vi "Handle Messages.vi"(8 "error in (no error)":errorcluster, 9 "Message Data":variant, 10 "Message":string, 11 "Thermal Chamber Controller In":refnum<class "Thermal Chamber Controller.lvclass">) -> (0 "error out":errorcluster, 3 "Thermal Chamber Controller Out":refnum<class "Thermal Chamber Controller.lvclass">)   [LabVIEW 2020, in "Thermal Chamber Controller.lvclass"]
uses:
  Thermal Chamber Controller.lvclass
  C:/Program Files (x86)/National Instruments/LabVIEW 2020/vi.lib/Astemes/Triarc Framework/Helper Loop/Helper Loop.lvclass
  C:/Program Files (x86)/National Instruments/LabVIEW 2020/vi.lib/Astemes/Triarc Framework/Process/Process.lvclass
  <vilib>/Astemes/Triarc Framework/Process/Process.lvclass/Process.ctl
  Thermal Chamber Controller.lvclass/Thermal Chamber Controller.ctl
  Thermal Chamber Response Simlator/Thermal Chamber Response Simlator.lvclass/Thermal Chamber Response Simlator.ctl
  Private/Heater State.ctl
  <vilib>/Astemes/Triarc Framework/Process/Public/Lifecycle/Get Lifecycle State.vi
  <vilib>/Astemes/Triarc Framework/Process/Public/Broadcasting/Register for Broadcast Events.vi
  <vilib>/Astemes/Triarc Framework/Broadcast Event Helpers/Dequeue Broadcast Message by Message.vi
  <vilib>/Astemes/Triarc Framework/Process/Private/SubVIs/Handle Debug Data.vi
  <vilib>/Utility/error.llb/Clear Errors.vi
  <vilib>/Astemes/Triarc Framework/Broadcast Event Helpers/Execution timer.vi
  <vilib>/Utility/High Resolution Relative Seconds.vi
  <vilib>/Utility/error.llb/Error Cluster From Error Code.vi
  <vilib>/Astemes/Triarc Framework/Broadcast Event Helpers/Dequeue Broadcast Message.vi
  Thermal Chamber Response Simlator/Private/Get Current Time if Not Set.vi
  Thermal Chamber Response Simlator/Get Actual Temperature.vi
  <vilib>/Astemes/Triarc Framework/Process/Process.lvclass
  <vilib>/Astemes/Triarc Framework/View/View.lvclass
  <vilib>/Astemes/Triarc Framework/Helper Loop/Helper Loop.lvclass
  Thermal Chamber Response Simlator/Thermal Chamber Response Simlator.lvclass
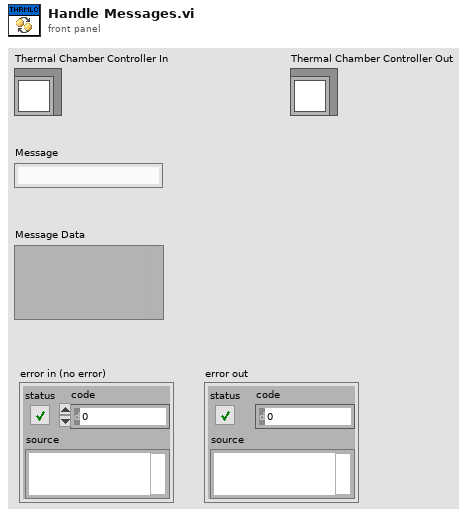
[diagram p1: front panel]
types:
  T1 = typedef "Thermal Chamber Controller.lvclass/Heater State.ctl" = enum16{"Heater Disabled", "Heater Enabled"}
  T2 = typedef "Thermal Chamber Controller.lvclass/Chamber State.ctl" = cluster{"Actual Temperature":dbl, "Temperature Set Point":dbl, "Temperature Ramp Rate":dbl, "Heater State":T1}
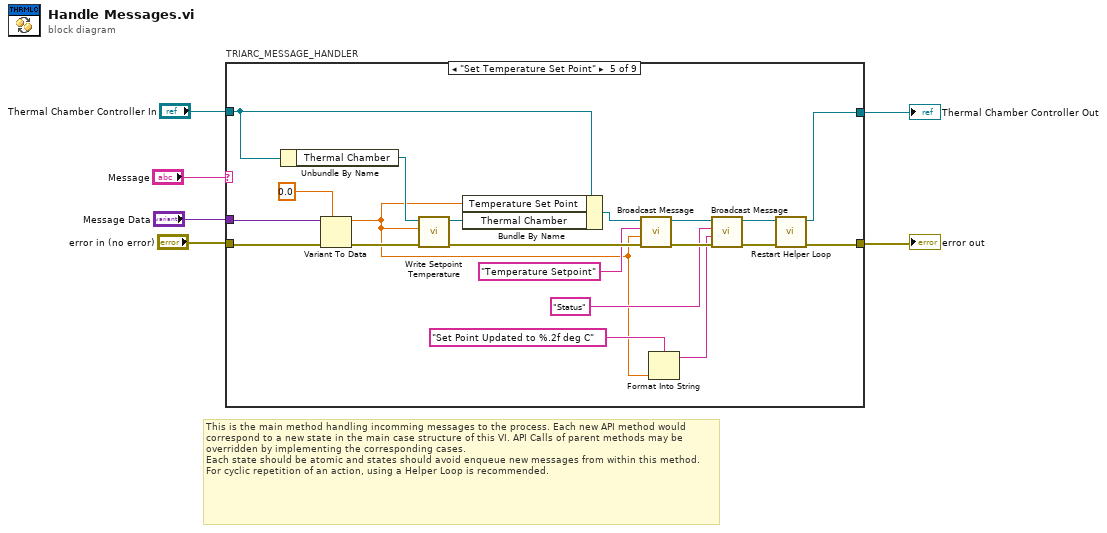
[diagram p0: block diagram]
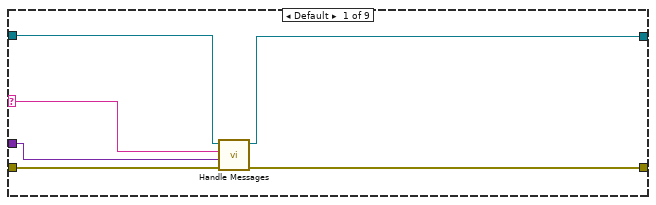
[diagram p2: hidden frame]
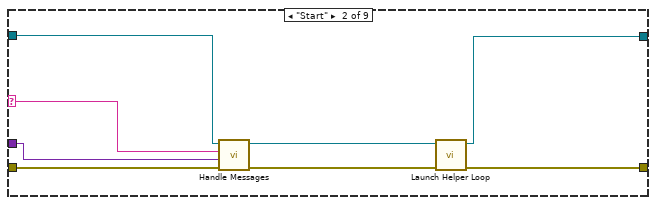
[diagram p3: hidden frame]
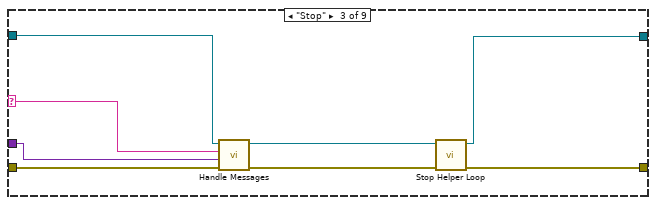
[diagram p4: hidden frame]
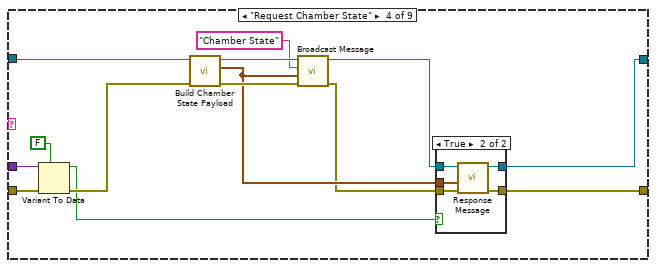
[diagram p5: hidden frame]
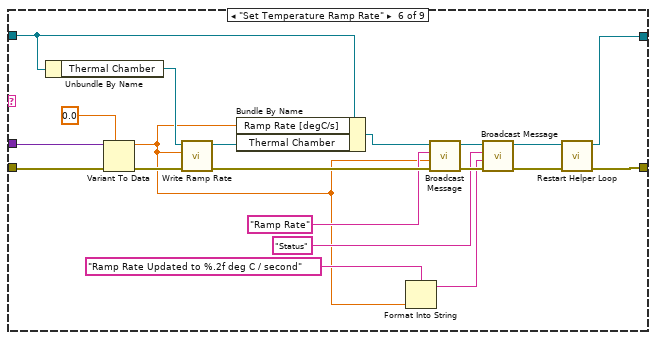
[diagram p7: hidden frame]
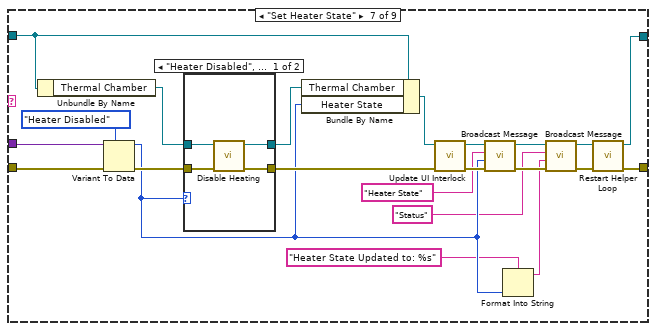
[diagram p8: hidden frame]
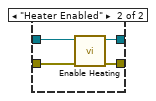
[diagram p9: hidden frame]
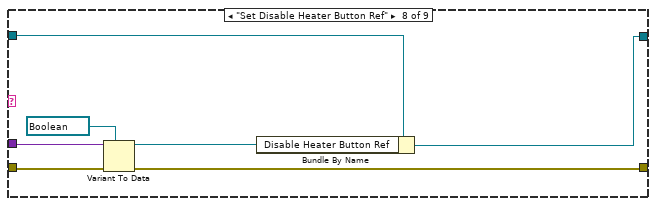
[diagram p10: hidden frame]
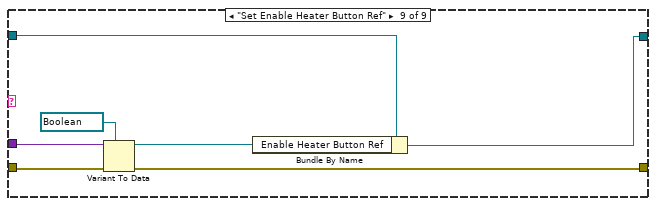
[diagram p11: hidden frame]
diagram:
  # "This is the main method handling incomming messages to the process. Each new API method would correspond to a new state in the main case structure of this VI. API Calls of parent methods may be overridden by implementing the corresponding cases.\nEach state should be atomic and states should avoid enqueue new messages from within this method. For cyclic repetition of an action, using a Helper Loop is recommended."
  n1 = case "TRIARC_MESSAGE_HANDLER" shown="\"Set Temperature Set Point\"" "Message" {
    selector: "Message" -> [w10 w18 w26 _ _ _ _ _ _]
    tunnel: "error in (no error)" -> [w9 w17 w25 w42 w69 w89 w111 w126 w133]
    tunnel: "Thermal Chamber Controller In" -> [w12 w20 w28 w37 w65 w86 w107 w125 w132]
    tunnel: "Message Data" -> [w11 w19 w27 w41 w67 w88 w109 w122 w128]
    tunnel: [w8 w13 w21 w39 w52 w72 w92 w123 w130] -> w2
    tunnel: [w7 w15 w23 w38 w50 w70 w90 w124 w131] -> w1
    frame Default {
      n2 = call-parent "Handle Messages.vi"("error in (no error)"=w9, "Message Data"=w11, "Message"=w10, "View In"=w12) -> ("error out"=w8:errorcluster, "View Out"=w7:refnum<class "Thermal Chamber Controller.lvclass">)  [unwired: 6 in]
    }
    frame "Start" {
      n3 = call-parent "Handle Messages.vi"("error in (no error)"=w17, "Message Data"=w19, "Message"=w18, "View In"=w20) -> ("error out"=w14:errorcluster, "View Out"=w16:refnum<class "Thermal Chamber Controller.lvclass">)  [unwired: 6 in]
      n4 = call <vilib>:"Launch Helper Loop.vi"("error in (no error)"=w14, "Helper Loop In"=w16) -> ("error out"=w13:errorcluster, "Helper Loop Out"=w15:refnum<class "Thermal Chamber Controller.lvclass">)  [unwired: 8 in]
    }
    frame "Stop" {
      n5 = call-parent "Handle Messages.vi"("error in (no error)"=w25, "Message Data"=w27, "Message"=w26, "View In"=w28) -> ("error out"=w22:errorcluster, "View Out"=w24:refnum<class "Thermal Chamber Controller.lvclass">)  [unwired: 6 in]
      n6 = call <vilib>:"Stop Helper Loop.vi"("error in (no error)"=w22, "Helper Loop In"=w24) -> ("error out"=w21:errorcluster, "Helper Loop Out"=w23:refnum<class "Thermal Chamber Controller.lvclass">)  [unwired: 7 in, 1 out]
    }
    frame "Request Chamber State" {
      n7 = Variant To Data(error in=w42, type=FALSE, Variant=w41) -> (data=w31:bool, error out=w35:errorcluster)
      n8 = call "Build Chamber State Payload.vi"("error in (no error)"=w35, "Thermal Chamber Controller In"=w37) -> ("error out"=w36:errorcluster, "Chamber State Payload"=w32:T2, "Thermal Chamber Controller Out"=w34:refnum<class "Thermal Chamber Controller.lvclass">)  [unwired: 7 in]
      n9 = call-dynamic "Broadcast Message.vi"("error in (no error)"=w36, "Message Data"=w32, "Message"="Chamber State", "Process In"=w34) -> ("error out"=w29:errorcluster, "Process Out"=w30:refnum<class "Thermal Chamber Controller.lvclass">)  [unwired: 6 in]
      n10 = case shown="True" w31 {
        tunnel: [w43 w49] -> w39
        tunnel: [w44 w48] -> w38
        tunnel: w29 -> [w43 w47]
        tunnel: w30 -> [w44 w46]
        tunnel: w32 -> [_ w45]
        frame False {
        }
        frame True {
          n11 = call <vilib>:"Response Message.vi"("error in (no error)"=w47, "Response Message Data"=w45, "Process In"=w46) -> ("error out"=w49:errorcluster, "Process Out"=w48:refnum<class "Thermal Chamber Controller.lvclass">)  [unwired: 7 in]
        }
      }
    }
    frame "Set Temperature Set Point" {
      n12 = Unbundle By Name(w65) -> ("Thermal Chamber"=w63:refnum<class "Thermal Chamber Response Simlator.lvclass">)
      n13 = Variant To Data(error in=w69, type=0.0 ("Numeric"), Variant=w67) -> (data=w54:dbl, error out=w68:errorcluster)
      n14 = call "Write Setpoint Temperature.vi"("error in (no error)"=w68, "Setpoint Temperature [degC]"=w54, "Thermal Chamber Response Simlator In"=w63) -> ("error out"=w64:errorcluster, "Thermal Chamber Response Simlator Out"=w62:refnum<class "Thermal Chamber Response Simlator.lvclass">)  [unwired: 7 in]
      n15 = Bundle By Name(cluster=w65, "Temperature Set Point"=w54, "Thermal Chamber"=w62) -> (w60:refnum<class "Thermal Chamber Controller.lvclass">)
      n16 = call-dynamic "Broadcast Message.vi"("error in (no error)"=w64, "Message Data"=w54, "Message"="Temperature Setpoint", "Process In"=w60) -> ("error out"=w61:errorcluster, "Process Out"=w57:refnum<class "Thermal Chamber Controller.lvclass">)  [unwired: 6 in]
      n17 = Format Into String(format string="Set Point Updated to %.2f deg C", w54) -> (resulting string=w53:string)  [unwired: 2 in, 1 out]
      n18 = call-dynamic "Broadcast Message.vi"("error in (no error)"=w61, "Message Data"=w53, "Message"="Status", "Process In"=w57) -> ("error out"=w58:errorcluster, "Process Out"=w51:refnum<class "Thermal Chamber Controller.lvclass">)  [unwired: 6 in]
      n19 = call "Restart Helper Loop.vi"("error in (no error)"=w58, "Thermal Chamber Controller In"=w51) -> ("error out"=w52:errorcluster, "Thermal Chamber Controller Out"=w50:refnum<class "Thermal Chamber Controller.lvclass">)  [unwired: 8 in]
    }
    frame "Set Temperature Ramp Rate" {
      n20 = Unbundle By Name(w86) -> ("Thermal Chamber"=w82:refnum<class "Thermal Chamber Response Simlator.lvclass">)
      n21 = Variant To Data(error in=w89, type=0.0 ("Numeric"), Variant=w88) -> (data=w73:dbl, error out=w85:errorcluster)
      n22 = call "Write Ramp Rate.vi"("error in (no error)"=w85, "Ramp Rate [degC/s]"=w73, "Thermal Chamber Response Simlator In"=w82) -> ("error out"=w84:errorcluster, "Thermal Chamber Response Simlator Out"=w83:refnum<class "Thermal Chamber Response Simlator.lvclass">)  [unwired: 7 in]
      n23 = Bundle By Name(cluster=w86, "Ramp Rate [degC/s]"=w73, "Thermal Chamber"=w83) -> (w80:refnum<class "Thermal Chamber Controller.lvclass">)
      n24 = Format Into String(format string="Ramp Rate Updated to %.2f deg C / second", w73) -> (resulting string=w74:string)  [unwired: 2 in, 1 out]
      n25 = call-dynamic "Broadcast Message.vi"("error in (no error)"=w84, "Message Data"=w73, "Message"="Ramp Rate", "Process In"=w80) -> ("error out"=w81:errorcluster, "Process Out"=w76:refnum<class "Thermal Chamber Controller.lvclass">)  [unwired: 6 in]
      n26 = call-dynamic "Broadcast Message.vi"("error in (no error)"=w81, "Message Data"=w74, "Message"="Status", "Process In"=w76) -> ("error out"=w77:errorcluster, "Process Out"=w71:refnum<class "Thermal Chamber Controller.lvclass">)  [unwired: 6 in]
      n27 = call "Restart Helper Loop.vi"("error in (no error)"=w77, "Thermal Chamber Controller In"=w71) -> ("error out"=w72:errorcluster, "Thermal Chamber Controller Out"=w70:refnum<class "Thermal Chamber Controller.lvclass">)  [unwired: 8 in]
    }
    frame "Set Heater State" {
      n28 = Unbundle By Name(w107) -> ("Thermal Chamber"=w105:refnum<class "Thermal Chamber Response Simlator.lvclass">)
      n29 = Variant To Data(error in=w111, type=Heater_State."Heater Disabled" ("Heater State"), Variant=w109) -> (data=w98:T1, error out=w110:errorcluster)
      n30 = case shown="\"Heater Disabled\", Default" w98 {
        tunnel: w110 -> [w115 w119]
        tunnel: [w114 w118] -> w106
        tunnel: w105 -> [w113 w117]
        tunnel: [w112 w116] -> w104
        frame "Heater Disabled", Default {
          n31 = call "Disable Heating.vi"("error in (no error)"=w115, "Thermal Chamber Response Simlator In"=w113) -> ("error out"=w114:errorcluster, "Thermal Chamber Response Simlator Out"=w112:refnum<class "Thermal Chamber Response Simlator.lvclass">)  [unwired: 8 in]
        }
        frame "Heater Enabled" {
          n32 = call "Enable Heating.vi"("error in (no error)"=w119, "Thermal Chamber Response Simlator In"=w117) -> ("error out"=w118:errorcluster, "Thermal Chamber Response Simlator Out"=w116:refnum<class "Thermal Chamber Response Simlator.lvclass">)  [unwired: 8 in]
        }
      }
      n33 = Bundle By Name(cluster=w107, "Thermal Chamber"=w104, "Heater State"=w98) -> (w102:refnum<class "Thermal Chamber Controller.lvclass">)
      n34 = call "Update UI Interlock.vi"("error in (no error)"=w106, "Thermal Chamber Controller In"=w102) -> ("error out"=w103:errorcluster, "Thermal Chamber Controller Out"=w99:refnum<class "Thermal Chamber Controller.lvclass">)  [unwired: 8 in]
      n35 = call-dynamic "Broadcast Message.vi"("error in (no error)"=w103, "Message Data"=w98, "Message"="Heater State", "Process In"=w99) -> ("error out"=w101:errorcluster, "Process Out"=w95:refnum<class "Thermal Chamber Controller.lvclass">)  [unwired: 6 in]
      n36 = Format Into String(format string="Heater State Updated to: %s", w98) -> (resulting string=w93:string)  [unwired: 2 in, 1 out]
      n37 = call-dynamic "Broadcast Message.vi"("error in (no error)"=w101, "Message Data"=w93, "Message"="Status", "Process In"=w95) -> ("error out"=w96:errorcluster, "Process Out"=w91:refnum<class "Thermal Chamber Controller.lvclass">)  [unwired: 6 in]
      n38 = call "Restart Helper Loop.vi"("error in (no error)"=w96, "Thermal Chamber Controller In"=w91) -> ("error out"=w92:errorcluster, "Thermal Chamber Controller Out"=w90:refnum<class "Thermal Chamber Controller.lvclass">)  [unwired: 8 in]
    }
    frame "Set Disable Heater Button Ref" {
      n39 = Variant To Data(error in=w126, type=refnum<vi> refnum ("Disable Heater Button Ref"), Variant=w122) -> (data=w120:refnum<vi>, error out=w123:errorcluster)
      n40 = Bundle By Name(cluster=w125, "Disable Heater Button Ref"=w120) -> (w124:refnum<class "Thermal Chamber Controller.lvclass">)
    }
    frame "Set Enable Heater Button Ref" {
      n41 = Variant To Data(error in=w133, type=refnum<vi> refnum ("Disable Heater Button Ref"), Variant=w128) -> (data=w129:refnum<vi>, error out=w130:errorcluster)
      n42 = Bundle By Name(cluster=w132, "Enable Heater Button Ref"=w129) -> (w131:refnum<class "Thermal Chamber Controller.lvclass">)
    }
  }
  "error out" <- w2
  "Thermal Chamber Controller Out" <- w1
